vi "change file suffix.vi"(8 "File root suffix":string, 9 "File suffix":string, 11 "Path":path) -> (3 "Path with different file suffix":path)   [LabVIEW 2017]
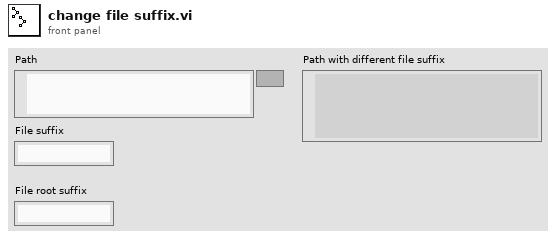
[diagram p1: front panel]
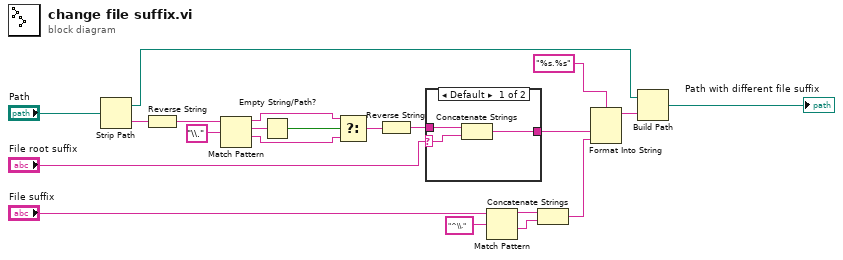
[diagram p0: block diagram]
diagram:
  n1 = Strip Path(path="Path") -> (stripped path=w16:path, name=w21:string)
  n2 = Reverse String(1:w21) -> (0:w20:string)
  n3 = Match Pattern(string=w20, regular expression="\\.") -> (before substring=w5:string, match substring=w4:string, after substring=w1:string)  [unwired: 1 in, 1 out]
  n4 = Empty String/Path?(string/path=w4) -> (empty?=w2:bool)
  n5 = Select(t=w5, s=w2, f=w1) -> (s? t:f=w3:string)
  n6 = Reverse String(1:w3) -> (0:w7:string)
  n7 = case shown="Default" "File root suffix" {
    selector: "File root suffix" -> [w23 _]
    tunnel: [w22 w25] -> w6
    tunnel: w7 -> [w24 w25]
    frame Default {
      n8 = Concatenate Strings(w24, w23) -> (w22:string)
    }
    frame "" {
    }
  }
  n9 = Match Pattern(string="File suffix", regular expression="^\\.") -> (before substring=w11:string, after substring=w10:string)  [unwired: 1 in, 2 out]
  n10 = Concatenate Strings(w11, w10) -> (w9:string)
  n11 = Format Into String(format string="%s.%s", w6, w9) -> (resulting string=w17:string)  [unwired: 2 in, 1 out]
  n12 = Build Path(base path=w16, name or relative path=w17) -> (appended path=→"Path with different file suffix":path)
